vi "PatternMatchInitialize.vi"(8 "Error In":errorcluster, 11 "script path":string[](array[string])=["C:\\Users\\user\\Desktop\\iVision_20160424_Caliper_Coor -Cal\\Data\\up", "C:\\Users\\user\\Desktop\\iVision_20160424_Caliper_Coor -Cal\\Data\\down"]) -> (0 "Error Out":errorcluster)   [LabVIEW 2015]
uses:
  Controls/Vision_DataEntry.ctl
  Process/Controls/Process_Setting.ctl
  Process/Controls/Process_Type.ctl
  Analysis/Controls/Analysis_Setting.ctl
  Analysis/Controls/Analysis_Type.ctl
  Caliper/Controls/CaliperDataEntry.ctl
  Caliper/Controls/CaliperType.ctl
  Caliper/Controls/SelectionListEntry.ctl
  Caliper/Controls/SelectionListEntryPointType.ctl
  Caliper/Controls/CaliperResult.ctl
  Coordinate/Control/CoordinatteEntry.ctl
  Coordinate/Control/CoordinateAnalysisSetting.ctl
  Coordinate/Control/CoordinateCaliperSetting.ctl
  Controls/ParameterData.ctl
  <vilib>/vision/Image Controls.llb/IMAQ Image.ctl
  Controls/iVisionSEQ.ctl
  Analysis/Controls/Parttern Match/Analysis_PatternMatch_Parameter.ctl
  [Global] CoordTemp.vi
  [Global] Template.vi
  [Global] RootPath.vi
  [Global]CalTemp.vi
panel:
  in  "output cluster":T16 {"All ROI"."Analysis_Setting"."Analysis_Type" items=["None", "PatternMatch", "Edge Detection", "Barcode 1D", "Barcode 2D", "Clamp", "Clamp MAX", "Particle", "Histogram", "Straight Edge", "Circle", "Shape Detect", "OCR", "Contour", "ColorMatch"]; "AllCaliperEntries"."CaliperType" items=["Distance", "Mid Point", "Perpendicular Projection", "Lines Intersection", "Angle from Horizontal", "Angle from Vertical", "Angle Defined by 3 Points", "Angle Defined by 4 Points", "Bissecting Line", "Mid Line", "Center of Mass", "Area", "Line Fit", "Circle Fit", "Ellipse Fit"]; "CoordinatteEntry Output"."CaliperSetting"."CaliperEntry"."CaliperType" items=["Distance", "Mid Point", "Perpendicular Projection", "Lines Intersection", "Angle from Horizontal", "Angle from Vertical", "Angle Defined by 3 Points", "Angle Defined by 4 Points", "Bissecting Line", "Mid Line", "Center of Mass", "Area", "Line Fit", "Circle Fit", "Ellipse Fit"]; "CoordinatteEntry Output"."OriginPointInfo"."Mode" items=["Horizontal Motion", "Vertical Motion", "Horizontal and Vertical Motion", "Horizontal. Vertical and Angular Motion"]; "CoordinatteEntry Output"."AnalysisSetting"."ROI"."Contours"."Type" items=["No Selection", "Point", "Line", "Rectangle", "Oval", "Polygon", "Freehand Region", "Annulus", "Unused2", "Unused3", "Broken Line", "Freehand Line", "Rotated Rectangle"]; "AllCaliperEntries"."CaliperType" items=["Distance", "Mid Point", "Perpendicular Projection", "Lines Intersection", "Angle from Horizontal", "Angle from Vertical", "Angle Defined by 3 Points", "Angle Defined by 4 Points", "Bissecting Line", "Mid Line", "Center of Mass", "Area", "Line Fit", "Circle Fit", "Ellipse Fit"]}
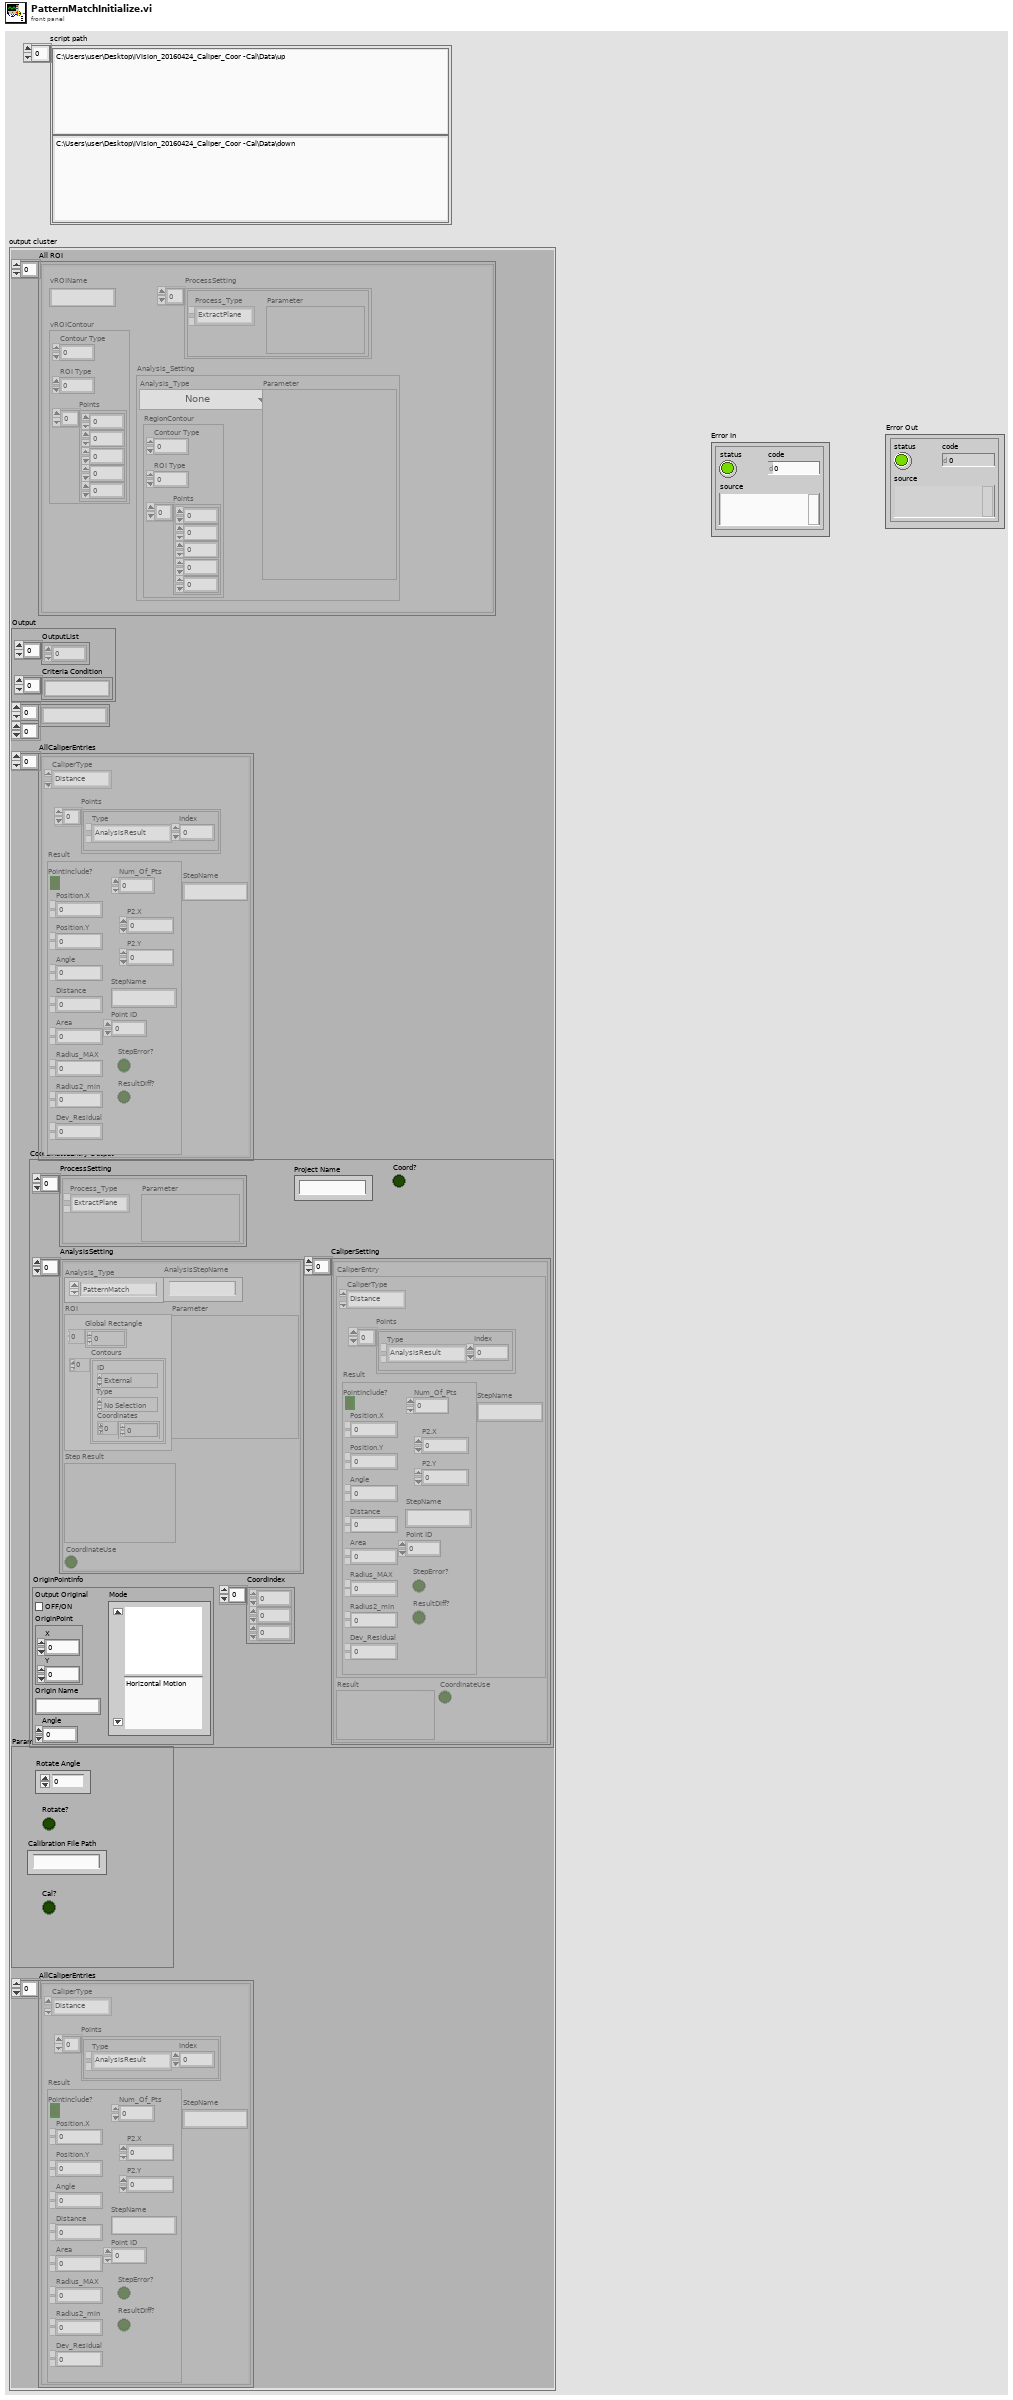
[diagram p1: front panel]
types:
  T1 = typedef "Vision_DataEntry.ctl" = cluster{"vROIName":string, "vROIContour":cluster{"Contour Type":u32, "ROI Type":u32, "Points":i32[]}, "ProcessSetting":T2[], "Analysis_Setting":T4}
  T2 = typedef "Process_Setting.ctl" = cluster{"Process_Type":T3, "Parameter":variant}
  T3 = typedef "Process_Type.ctl" = enum16{"None", "ExtractPlane", "BinaryMono", "Operators", "GrayMorphology", "Filters", "Lookup Table", "Particle Filter", "Mask"}
  T4 = typedef "Analysis_Setting.ctl" = cluster{"Analysis_Type":T5, "RegionContour":cluster{"Contour Type":u32, "ROI Type":u32, "Points":i32[]}, "Parameter":variant}
  T5 = typedef "Analysis_Type.ctl" = u16
  T6 = typedef "CaliperDataEntry.ctl" = cluster{"CaliperType":T7, "Points":T8[], "Result":T10, "StepName":string}
  T7 = typedef "CaliperType.ctl" = u32
  T8 = typedef "SelectionListEntry.ctl" = cluster{"Type":T9, "Index":i32}
  T9 = typedef "SelectionListEntryPointType.ctl" = enum16{"AnalysisResult", "CaliperResult"}
  T10 = typedef "CaliperResult.ctl" = cluster{"PointInclude?":bool, "Num_Of_Pts":u8, "Position.X":dbl, "Position.Y":dbl, "Angle":dbl, "Distance":dbl, "Area":dbl, "Radius_MAX":dbl, "Radius2_min":dbl, "Dev_Residual":dbl, "P2.X":dbl, "P2.Y":dbl, "StepName":string, "Point ID":u8, "StepError?":bool, "ResultDiff?":bool}
  T11 = typedef "CoordinatteEntry.ctl" = cluster{"ProcessSetting":T2[], "Project Name":string, "AnalysisSetting":T12[], "Coord?":bool, "OriginPointInfo":cluster{"Output Original":bool, "Origin Name":string, "Angle":dbl, "Mode":u16, "OriginPoint":cluster{"X":dbl, "Y":dbl}}, "CaliperSetting":T14[], "CoordIndex":i32[]}
  T12 = typedef "CoordinateAnalysisSetting.ctl" = cluster{"Analysis_Type":enum16{"PatternMatch", "Straight Edge"}, "ROI ":T13, "Parameter":variant, "Step Result":variant, "AnalysisStepName":string, "CoordinateUse":bool}
  T13 = typedef "ROI Descriptor" = cluster{"Global Rectangle":i32[], "Contours":cluster{"ID":enum32{"External", "Internal"}, "Type":u32, "Coordinates":i32[]}[]}
  T14 = typedef "CoordinateCaliperSetting.ctl" = cluster{"Result":variant, "CoordinateUse":bool, "CaliperEntry":T6}
  T15 = typedef "ParameterData.ctl" = cluster{"Rotate Angle":dbl, "Rotate?":bool, "Calibration File Path":string, "Cal?":bool}
  T16 = cluster{"All ROI":T1[], "Output":cluster{"OutputList":u16[], "Criteria Condition":string[]}, string[][], "AllCaliperEntries":T6[], "CoordinatteEntry Output":T11, "ParameterData Out":T15, "AllCaliperEntries":T6[]}
  T17 = typedef "IMAQ Image.ctl" = refnum<image>
  T18 = cluster{"Script Name":string, "TemplateArray":cluster{"ROI Name":string, "TemplateImage":T17}[]}[]
  T19 = typedef "iVisionSEQ.ctl" = cluster{"iVision_Version":string, "iVisionSEQParam":variant}
  T20 = enum16{"open", "replace", "create", "open or create", "replace or create", "replace or create with confirmation"}
  T21 = cluster{"All ROI":cluster{"vROIName":string, "vROIContour":cluster{"Contour Type":u32, "ROI Type":u32, "Points":i32[]}, "ProcessSetting":cluster{"Process_Type":enum16{"None", "ExtractPlane", "BinaryMono", "Operators", "GrayMorphology", "Filters", "Lookup Table", "Particle Filter", "Mask"}, "Parameter":variant}[], "Analysis_Setting":cluster{"Analysis_Type":enum16{"None", "PatternMatch", "Edge Detection", "Barcode 1D", "Barcode 2D", "Clamp", "Clamp MAX", "Particle", "Histogram", "Straight Edge", "Circle", "Shape Dectect", "OCR"}, "RegionContour":cluster{"Contour Type":u32, "ROI Type":u32, "Points":i32[]}, "Parameter":variant}}[], "Output":cluster{"OutputList":u16[], "Criteria Condition":string[]}, string[][], "AllCaliperEntries":cluster{"CaliperType":u32, "Points":cluster{"Type":enum16{"AnalysisResult", "CaliperResult"}, "Index":i32}[], "Result":cluster{"PointInclude?":bool, "Num_Of_Pts":u8, "Position.X":dbl, "Position.Y":dbl, "Angle":dbl, "Distance":dbl, "Area":dbl, "Radius_MAX":dbl, "Radius2_min":dbl, "Dev_Residual":dbl, "P2.X":dbl, "P2.Y":dbl, "StepName":string, "Point ID":u8, "StepError?":bool, "ResultDiff?":bool}, "StepName":string}[], "CoordinatteEntry Output":cluster{"ProcessSetting":cluster{"Process_Type":enum16{"None", "ExtractPlane", "BinaryMono", "Operators", "GrayMorphology", "Filters", "Lookup Table", "Particle Filter", "Mask"}, "Parameter":variant}[], "Project Name":string, "AnalysisSetting":cluster{"Analysis_Type":enum16{"PatternMatch", "Straight Edge"}, "ROI ":T13, "Parameter":variant, "Step Result":variant, "OriginPointInfo":cluster{"Output Original":bool, "Origin Name":string, "Angle":dbl, "Mode":u16, "OriginPoint":cluster{"X":dbl, "Y":dbl}}, "AnalysisStepName":string}[], "Coord?":bool}, "ParameterData Out":cluster{"Rotate Angle":dbl, "Rotate?":bool, "Calibration File Path":string, "Cal?":bool}, "AllCaliperEntries":cluster{"CaliperType":u32, "Points":cluster{"Type":enum16{"AnalysisResult", "CaliperResult"}, "Index":i32}[], "Result":cluster{"PointInclude?":bool, "Num_Of_Pts":u8, "Position.X":dbl, "Position.Y":dbl, "Angle":dbl, "Distance":dbl, "Area":dbl, "Radius_MAX":dbl, "Radius2_min":dbl, "Dev_Residual":dbl, "P2.X":dbl, "P2.Y":dbl, "StepName":string, "Point ID":u8, "StepError?":bool, "ResultDiff?":bool}, "StepName":string}[]}
  T22 = cluster{"Algorithm":i32, "Match Parameters":cluster{"Number of Matches Requested":i32, "Minimum Match Score":sgl, "Angle Ranges":cluster{"Start Angle":sgl, "End Angle":sgl}[]}, "ROI Descriptor":T13, "Advanced Options":cluster{"Item":u16, "Value":dbl}[], "Template path":string}
  T23 = cluster{"Script Name":string, "TemplateArray":cluster{"ROI Name":string, "TemplateImage":T17}[]}
  T24 = cluster{"ROI Name":string, "TemplateImage":T17}[]
  T25 = typedef "Analysis_PatternMatch_Parameter.ctl" = cluster{"Algorithm":i32, "Match Parameters":cluster{"Number of Matches Requested":i32, "Minimum Match Score":sgl, "Angle Ranges":cluster{"Start Angle":sgl, "End Angle":sgl}[]}, "ROI Descriptor":T13, "Advanced Options":cluster{"Item":u16, "Value":dbl}[], "Template path":string, "XOffset":i32, "YOffset":i32}
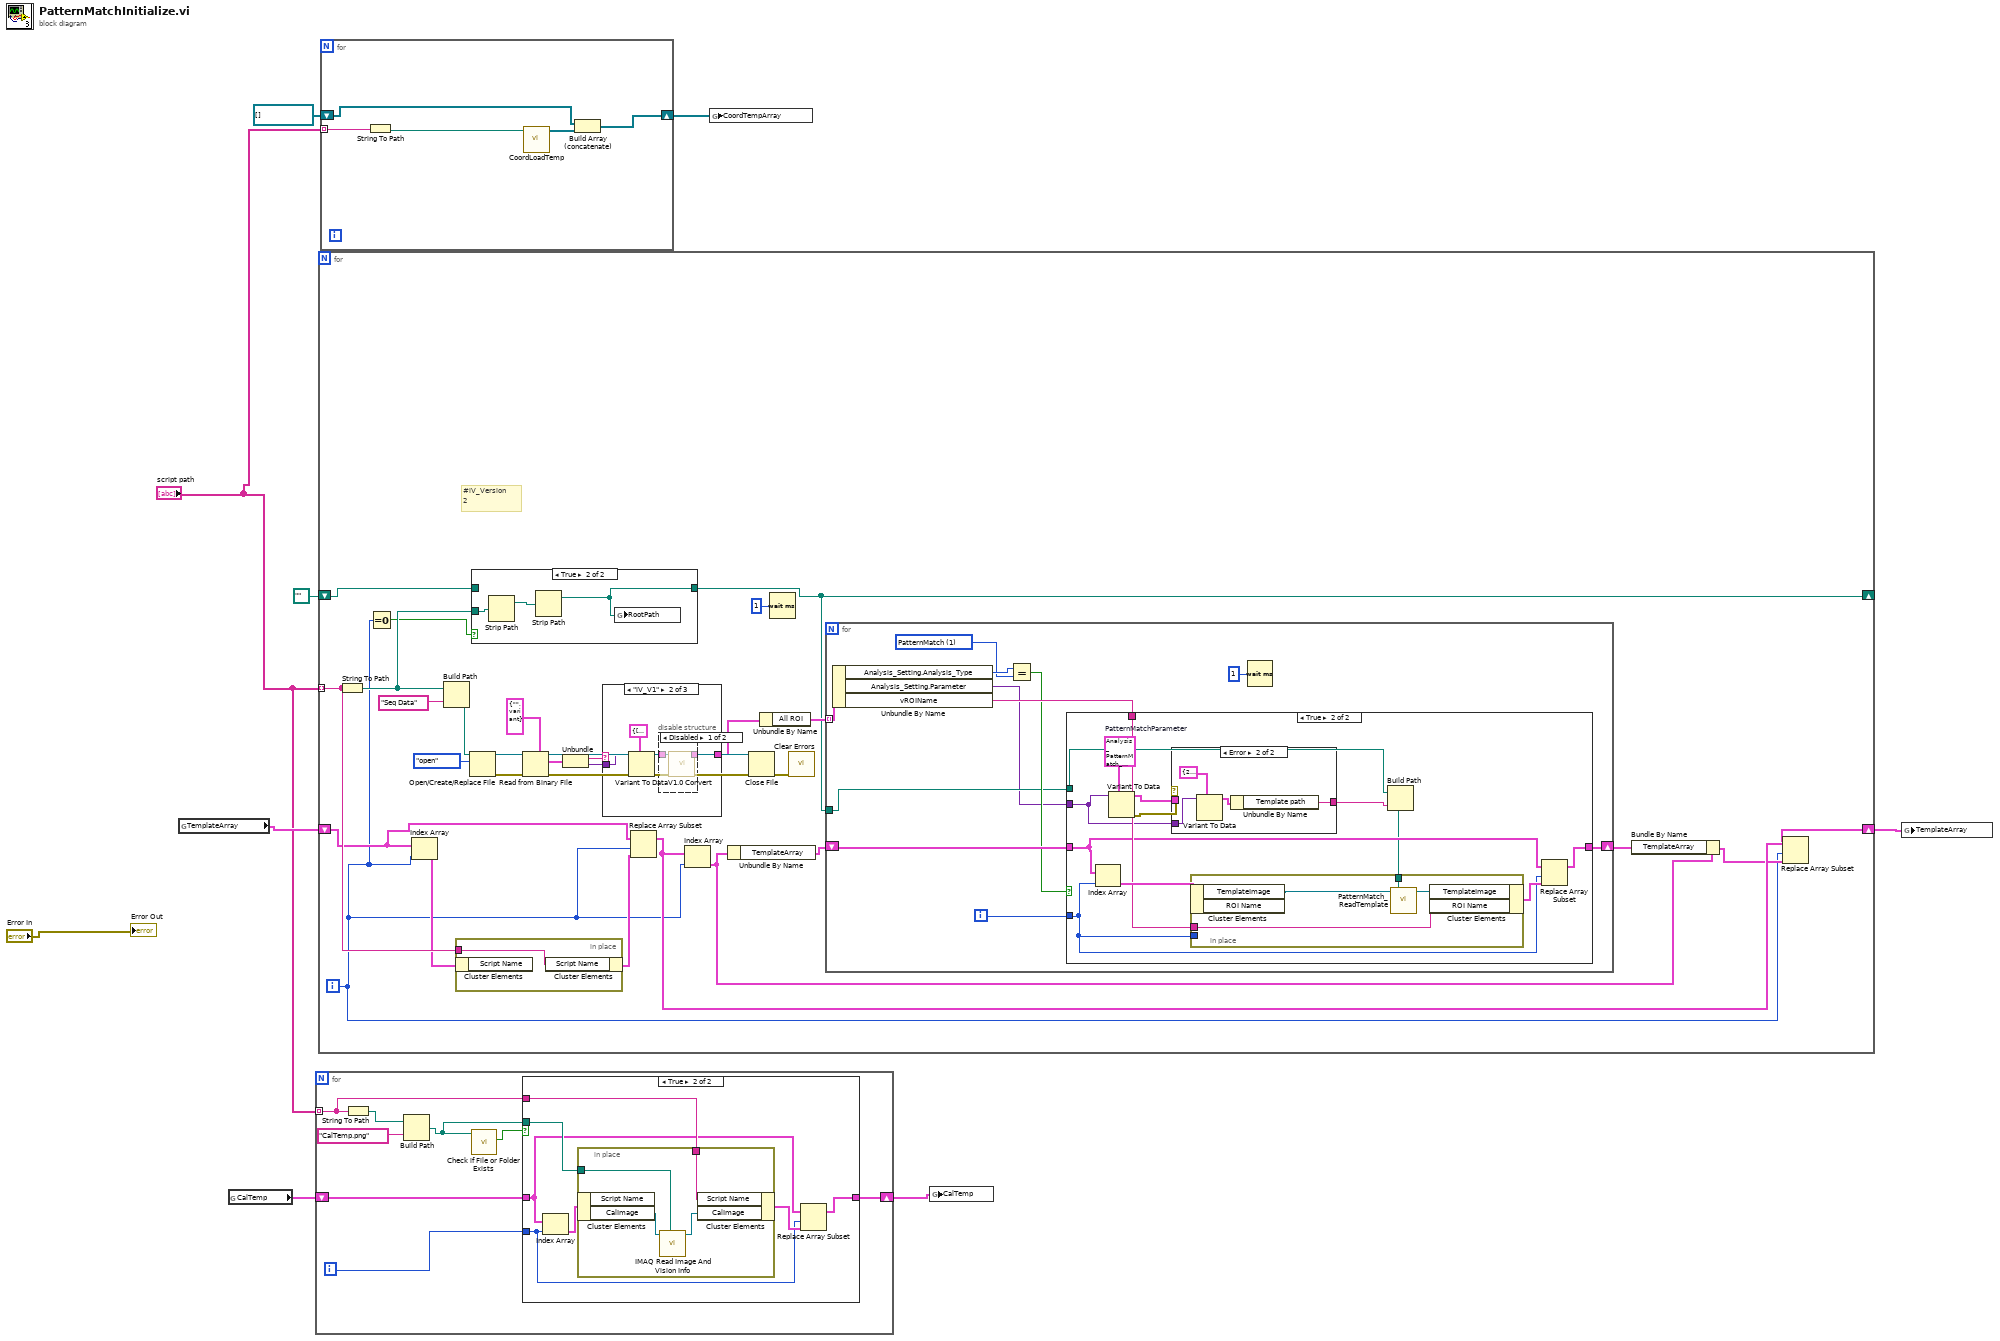
[diagram p0: block diagram]
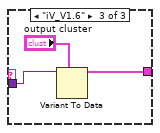
[diagram p5: hidden frame]
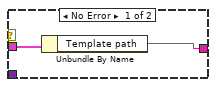
[diagram p8: hidden frame]
diagram:
  n1 = global read "[Global] Template.vi" "TemplateArray"() -> (w6:T18)
  n2 = global read "[Global]CalTemp.vi" "CalTemp"() -> (w5:cluster{"Script Name":string, "CalImage":T17}[])
  n3 = for {
    tunnel: "script path" -> [w11] mode=indexing
    shift-right: [w10] -> w4
    shift-left: w5 -> [w15]
    i -> [w13]
    n4 = String To Path(string=w11) -> (path=w16:path)
    n5 = Build Path(base path=w16, name or relative path="CalTemp.png") -> (appended path=w12:path)
    n6 = call <vilib>:"Check if File or Folder Exists.vi"("path"=w12) -> ("file or folder exists?"=w14:bool)  [unwired: 8 in, 2 out]
    n7 = case shown="True" w14 {
      tunnel: w15 -> [w18 w22]
      tunnel: w13 -> [_ w20]
      tunnel: w12 -> [_ w24]
      tunnel: w11 -> [_ w23]
      tunnel: [w18 w19] -> w10
      frame False {
      }
      frame True {
        n8 = Index Array(array=w22, index=w20) -> (element=w25:cluster{"Script Name":string, "CalImage":T17})
        n9 = in-place {
          in-place-border: w24 -> [w28]
          in-place-border: w23 -> [w26]
          n10 = in-place-cluster #1(w25) -> ("CalImage"=w29:T17)  [unwired: 1 out]
          n11 = call "IMAQ Read Image And Vision Info"("File Path"=w28, "Image"=w29) -> ("Image Out"=w27:T17)  [unwired: 7 in, 2 out]
          n12 = in-place-cluster #1("Script Name"=w26, "CalImage"=w27) -> (w21:cluster{"Script Name":string, "CalImage":T17})
        }
        n13 = Replace Array Subset(array=w22, new element=w21, index=w20) -> (w19:cluster{"Script Name":string, "CalImage":T17}[])
      }
    }
  }
  n14 = for {
    tunnel: "script path" -> [w49] mode=indexing
    shift-right: [w41] -> w8
    shift-left: w6 -> [w46]
    shift-right: [w31] -> _
    shift-left: path "" ("stripped path") -> [w37]
    i -> [w39]
    # "#iV_Version\n2"
    n15 = String To Path(string=w49) -> (path=w50:path)
    n16 = Equal To 0?(x=w39) -> (x = 0?=w38:bool)
    n17 = Index Array(array=w46, index=w39) -> (element=w48:T23)
    n18 = Build Path(base path=w50, name or relative path="Seq Data") -> (appended path=w53:path)
    n19 = in-place {
      in-place-border: w49 -> [w73]
      n20 = in-place-cluster #2(w48) -> ()  [unwired: 1 out]
      n21 = in-place-cluster #2("Script Name"=w73) -> (w47:T23)
    }
    n22 = Open/Create/Replace File(file path (use dialog)=w53, operation (0:open)=T20."open") -> (refnum out=w56:refnum<file>, error out=w59:errorcluster)  [unwired: 4 in, 1 out]
    n23 = case shown="True" w38 {
      tunnel: w50 -> [_ w72]
      tunnel: [w69 w70] -> w31
      tunnel: w37 -> [w69 _]
      frame False {
      }
      frame True {
        n24 = Strip Path(path=w72) -> (stripped path=w71:path)  [unwired: 1 out]
        n25 = Strip Path(path=w71) -> (stripped path=w70:path)  [unwired: 1 out]
        n26 = global write "[Global] RootPath.vi" "RootPath"(w70) -> ()
      }
    }
    n27 = Read from Binary File(5:T19 {"iVision_Version"="", "iVisionSEQParam"=variant} ("iVisionSEQ"), 8:w59, 11:w56) -> (0:w58:errorcluster, 2:w35:T19, 3:w55:refnum<file>)  [unwired: 3 in, 1 out]
    n28 = Unbundle(w35) -> ("iVision_Version"=w34:string, "iVisionSEQParam"=w32:variant)
    n29 = case shown="\"iV_V1\"" w34 {
      tunnel: [_ w61 w67] -> w33
      tunnel: w32 -> [_ w60 w66]
      frame "False", Default {
      }
      frame "iV_V1" {
        n30 = Variant To Data(type=T21 {"All ROI"=[], "Output"={"OutputList"=[], "Criteria Condition"=[]}, [], "AllCaliperEntries"=[], "CoordinatteEntry Output"={"ProcessSetting"=[], "Project Name"="", "AnalysisSetting"=[], "Coord?"=FALSE}, "ParameterData Out"={"Rotate Angle"=0.0, "Rotate?"=FALSE, "Calibration File Path"="", "Cal?"=FALSE}, "AllCaliperEntries"=[]} ("Old"), Variant=w60) -> (data=w63:T21)  [unwired: 1 in, 1 out]
        n31 = disable-structure shown="Disabled" {
          disable-tunnel: w63 -> [w65 _]
          disable-tunnel: [w64 _] -> w61
          frame Disabled {
            n32 = call "V1.0 Convert.vi"("Old"=w65) -> ("NewOut"=w64:T16)  [unwired: 10 in]
          }
          frame Enabled {
          }
        }
      }
      frame "iV_V1.6" {
        n33 = Variant To Data(type="output cluster", Variant=w66) -> (data=w67:T16)  [unwired: 1 in, 1 out]
      }
    }
    n34 = Replace Array Subset(array=w46, new element=w47, index=w39) -> (w45:T18)
    n35 = Index Array(array=w45, index=w39) -> (element=w44:T23)
    n36 = Unbundle By Name(w44) -> ("TemplateArray"=w51:T24)
    n37 = Close File(refnum=w55, error in=w58) -> (error out=w30:errorcluster)  [unwired: 1 out]
    n38 = Unbundle By Name(w33) -> ("All ROI"=w52:T1[])
    n39 = Wait (ms)(milliseconds to wait=u32 1) -> ()  [unwired: 1 out]
    n40 = call <vilib>:"Clear Errors.vi"("error in (no error)"=w30) -> ()  [unwired: 5 in, 2 out]
    n41 = for {
      tunnel: w52 -> [w84] mode=indexing
      shift-right: [w78] -> w43
      shift-left: w51 -> [w79]
      tunnel: w31 -> [w75]
      i -> [w80]
      w82 = T5 1 items=["None", "PatternMatch", "Edge Detection", "Barcode 1D", "Barcode 2D", "Clamp", "Clamp MAX", "Particle", "Histogram", "Straight Edge", "Circle", "Shape Detect", "OCR", "Contour", "ColorMatch"] ("y")
      n42 = Unbundle By Name(w84) -> ("Analysis_Setting.Analysis_Type"=w83:T5, "Analysis_Setting.Parameter"=w74:variant, "vROIName"=w81:string)
      n43 = Equal?(x=w83, y=w82) -> (x = y?=w77:bool)
      n44 = case shown="True" w77 {
        tunnel: w81 -> [_ w97]
        tunnel: w80 -> [_ w93]
        tunnel: w79 -> [w85 w95]
        tunnel: [w85 w94] -> w78
        tunnel: w75 -> [_ w90]
        tunnel: w74 -> [_ w87]
        frame False {
        }
        frame True {
          w92 = T25 {"Algorithm"=2, "Match Parameters"={"Number of Matches Requested"=1, "Minimum Match Score"=750.0, "Angle Ranges"=[]}, "ROI Descriptor"={"Global Rectangle"=[], "Contours"=[]}, "Advanced Options"=[{"Item"=1, "Value"=1.0}, {"Item"=103, "Value"=1.0}], "Template path"="", "XOffset"=0, "YOffset"=0}  # PatternMatchParameter
          n45 = Index Array(array=w95, index=w93) -> (element=w98:cluster{"ROI Name":string, "TemplateImage":T17})
          n46 = Variant To Data(type=w92, Variant=w87) -> (data=w88:T25, error out=w89:errorcluster)  [unwired: 1 in]
          n47 = case shown="Error" w89 {
            tunnel: w88 -> [w100 _]
            tunnel: w87 -> [_ w103]
            tunnel: [w99 w101] -> w86
            frame No Error {
              n48 = Unbundle By Name(w100) -> ("Template path"=w99:string)
            }
            frame Error {
              n49 = Variant To Data(type=T22 {"Algorithm"=2, "Match Parameters"={"Number of Matches Requested"=1, "Minimum Match Score"=750.0, "Angle Ranges"=[]}, "ROI Descriptor"={"Global Rectangle"=[], "Contours"=[]}, "Advanced Options"=[{"Item"=1, "Value"=1.0}, {"Item"=103, "Value"=1.0}], "Template path"=""} ("PatternMatchParameter"), Variant=w103) -> (data=w102:T22)  [unwired: 1 in, 1 out]
              n50 = Unbundle By Name(w102) -> ("Template path"=w101:string)
            }
          }
          n51 = Build Path(base path=w90, name or relative path=w86) -> (appended path=w91:path)
          n52 = in-place {
            in-place-border: w91 -> [w108]
            in-place-border: w97 -> [w106]
            in-place-border: w93 -> [_]
            n53 = in-place-cluster #3(w98) -> ("TemplateImage"=w107:T17)  [unwired: 1 out]
            n54 = call "PatternMatch_ReadTemplate.vi"("template path"=w108, "Template"=w107) -> ("Template Out"=w105:T17)  [unwired: 8 in, 1 out]
            n55 = in-place-cluster #3("TemplateImage"=w105, "ROI Name"=w106) -> (w96:cluster{"ROI Name":string, "TemplateImage":T17})
          }
          n56 = Replace Array Subset(array=w95, new element=w96, index=w93) -> (w94:T24)
        }
      }
      n57 = Wait (ms)(milliseconds to wait=u32 1) -> ()  [unwired: 1 out]
    }
    n58 = Bundle By Name(cluster=w44, "TemplateArray"=w43) -> (w42:T23)
    n59 = Replace Array Subset(array=w45, new element=w42, index=w39) -> (w41:T18)
  }
  n60 = for {
    tunnel: "script path" -> [w113] mode=indexing
    shift-right: [w110] -> w2
    shift-left: T17[] [] -> [w109]
    n61 = String To Path(string=w113) -> (path=w112:path)
    n62 = call "CoordLoadTemp.vi"("appended path"=w112) -> ("CoordTempOut"=w111:T17[])  [unwired: 10 in]
    n63 = Build Array (concatenate)(w109, w111) -> (w110:T17[])
  }
  n64 = global write "[Global] CoordTemp.vi" "CoordTempArray"(w2) -> ()
  n65 = global write "[Global]CalTemp.vi" "CalTemp"(w4) -> ()
  n66 = global write "[Global] Template.vi" "TemplateArray"(w8) -> ()
  "Error Out" <- "Error In"
